vi "Did Something.vi"(8 "error in":errorcluster, 10 "Did Something Msg":string, 11 "Module ID":i32=-1) -> (0 "error out":errorcluster)   [LabVIEW 2022 SP3, in "My Cloneable Module.lvlib"]
doc: "Send the Did Something event to any VI registered to listen to this module's broadcast events.\n_____\nBased on DQMH Project Template 7.0.1.1316."
uses:
  My Cloneable Module.lvlib
  Do Something Argument--cluster.ctl
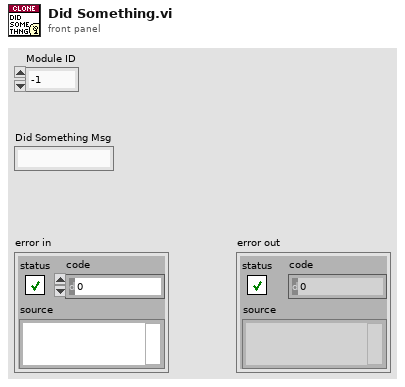
[diagram p1: front panel]
types:
  T1 = typedef "My Cloneable Module.lvlib/Do Something Argument--cluster.ctl" = cluster{"Module ID":i32, "Do Something Msg":string}
  T2 = typedef "My Cloneable Module.lvlib/Broadcast Events--cluster.ctl" = cluster{"Module Did Init":refnum<user-event>, "Status Updated":refnum<user-event>, "Error Reported":refnum<user-event>, "Did Something":refnum<user-event>, "Module Did Stop":refnum<user-event>, "Update Module Execution Status":refnum<user-event>}
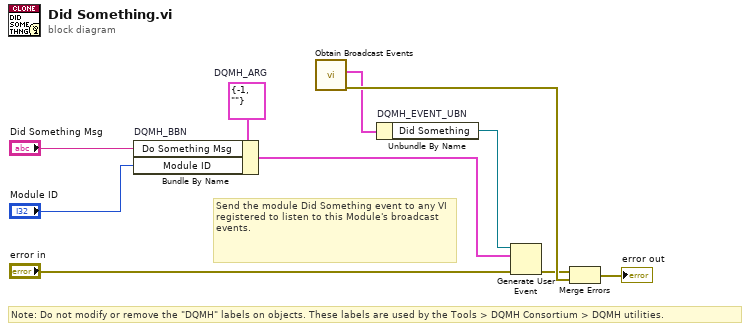
[diagram p0: block diagram]
diagram:
  w4 = T1 {"Module ID"=-1, "Do Something Msg"=""}  # DQMH_ARG
  # "Note: Do not modify or remove the \"DQMH\" labels on objects. These labels are used by the Tools > DQMH Consortium > DQMH utilities."
  # "Send the module Did Something event to any VI registered to listen to this Module's broadcast events."
  n1 = Bundle By Name "DQMH_BBN"(cluster=w4, "Do Something Msg"="Did Something Msg", "Module ID"="Module ID") -> (w3:T1)
  n2 = call "Obtain Broadcast Events.vi"() -> ("error out"=w8:errorcluster, "My Cloneable Module Broadcast Events"=w6:T2)  [unwired: 10 in]
  n3 = Unbundle By Name "DQMH_EVENT_UBN"(w6) -> ("Did Something"=w5:refnum<user-event>)
  n4 = Generate User Event(user event=w5, event data cluster=w3, error in="error in") -> (error out=w7:errorcluster)  [unwired: 1 in, 1 out]
  n5 = Merge Errors(w7, w8) -> (→"error out":errorcluster)
